vi "Load Config.vi"(8 "error in (no error)":errorcluster, 11 "HTTP Command Bridge in":refnum<class "HTTP Command Bridge.lvclass">) -> (0 "error out":errorcluster, 3 "HTTP Command Bridge out":refnum<class "HTTP Command Bridge.lvclass">)   [LabVIEW 2020, in "Volatus.lvlib" / "HTTP Command Bridge.lvclass"]
uses:
  HTTP Command Bridge.lvclass
  HTTP Command Bridge.lvclass/HTTP Command Bridge.ctl
  Module/Module.lvclass
  VolatusConfig/VolatusConfigElement/VolatusConfigElement.lvclass
  lv-cdm/CDM-Config/Config Element/Config Element.lvclass
  Command Dest.ctl
  MessageQ/MessageQ.lvclass
  Command Info.ctl
  C:/dev/lv20CE/relink/lv-volatus/Volatus/Module/Module.lvclass
  C:/dev/lv20CE/relink/lv-volatus/Volatus/HTTP Command Bridge/HTTP Command Bridge.lvclass
  VolatusConfig/Task/Task Config.lvclass
  C:/dev/lv20CE/relink/lv-volatus/VolatusConfig/VolatusConfigElement/VolatusConfigElement.lvclass
  C:/dev/lv20CE/relink/lv-volatus/VolatusConfig/Task/Task Config.lvclass
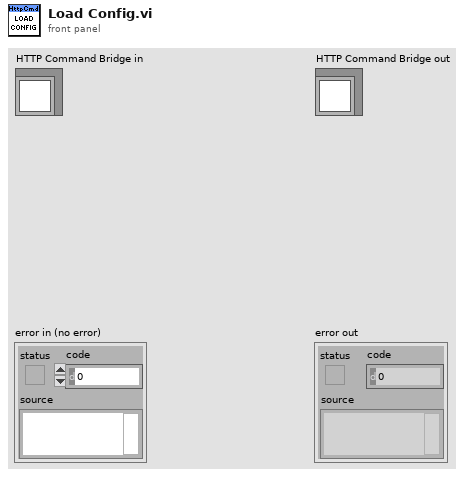
[diagram p1: front panel]
types:
  T1 = typedef "Volatus.lvlib/HTTP Command Bridge.lvclass/Command Info.ctl" = cluster{"Destination":T2, "Local Q":refnum<class "MessageQ.lvclass">, "Target":string, "Task":string}
  T2 = typedef "Volatus.lvlib/HTTP Command Bridge.lvclass/Command Dest.ctl" = enum16{"Local", "Remote"}
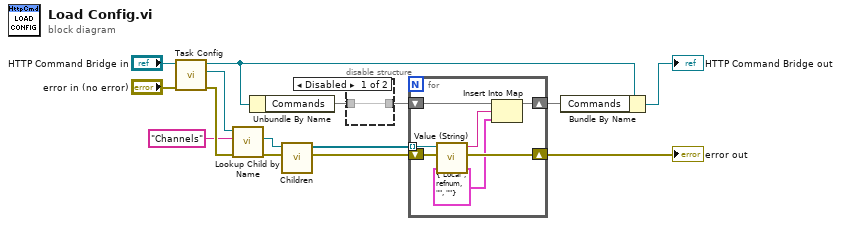
[diagram p0: block diagram]
diagram:
  n1 = call "Task Config.vi"("error in (no error)"="error in (no error)", "Module in"="HTTP Command Bridge in") -> ("error out"=w15:errorcluster, "Task Config"=w12:refnum<class "Task Config.lvclass">, "Module out"=w6:refnum<class "HTTP Command Bridge.lvclass">)  [unwired: 7 in]
  n2 = call "Lookup Child by Name.vi"("error in (no error)"=w15, "Child Name"="Channels", "VolatusConfigElement in"=w12) -> ("error out"=w9:errorcluster, "Child"=w10:refnum<class "Config Element.lvclass">)  [unwired: 5 in, 2 out]
  n3 = Unbundle By Name(w6) -> ("Commands"=w5:map{string, T1})
  n4 = call "Children.vi"("error in (no error)"=w9, "Config Element in"=w10) -> ("error out"=w7:errorcluster, "Elements"=w8:refnum<class "Config Element.lvclass">[])  [unwired: 8 in]
  n5 = disable-structure shown="Disabled" {
    disable-tunnel: w5 -> [w16 _]
    disable-tunnel: [w16 _] -> w4
    frame Disabled {
    }
    frame Enabled {
    }
  }
  n6 = for {
    tunnel: w8 -> [w23] mode=indexing
    shift-right: [w21] -> w1
    shift-left: w7 -> [w22]
    shift-right: [w17] -> w2
    shift-left: w4 -> [w20]
    n7 = call "Value (String).vi"("error in (no error)"=w22, "Config Element in"=w23) -> ("error out"=w21:errorcluster, "String Value"=w19:string)  [unwired: 8 in]
    n8 = Insert Into Map(map in=w20, key=w19, value=T1 {"Destination"=enum."Local", "Local Q"=refnum, "Target"="", "Task"=""}) -> (map out=w17:map{string, T1})  [unwired: 2 out]
  }
  "error out" <- w1
  n9 = Bundle By Name(cluster=w6, "Commands"=w2) -> (→"HTTP Command Bridge out":refnum<class "HTTP Command Bridge.lvclass">)
